vi "Команда обмена 5 (доп. команда) (SubVI).vi"(3 "Выстрелов до перемотки":u16=100, 7 "error in":errorcluster, 13 "номер мишени (id)":u16) -> (23 "Кластер параметров 15-ой команды":T1, 27 "error out":errorcluster)   [LabVIEW 2013]
doc: "Доп. команда - передача числа выстрелов до перемотки пленки"
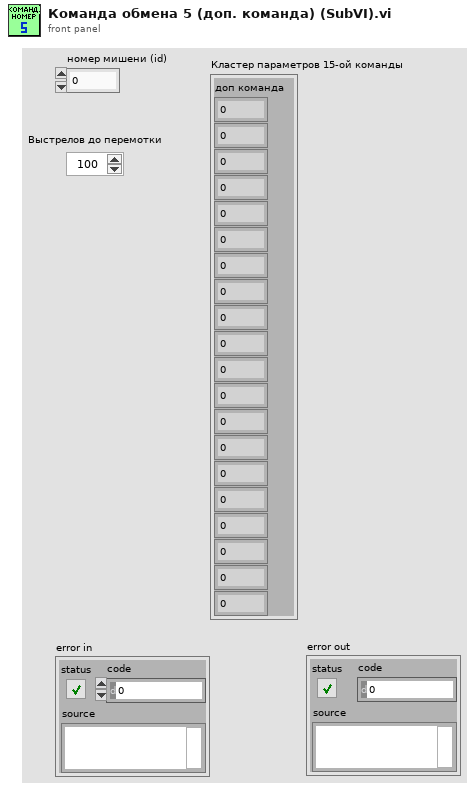
[diagram p1: front panel]
types:
  T1 = cluster{"доп команда":u8, u8, u8, u8, u8, u8, u8, u8, u8, u8, u8, u8, u8, u8, u8, u8, u8, u8, u8, u8}
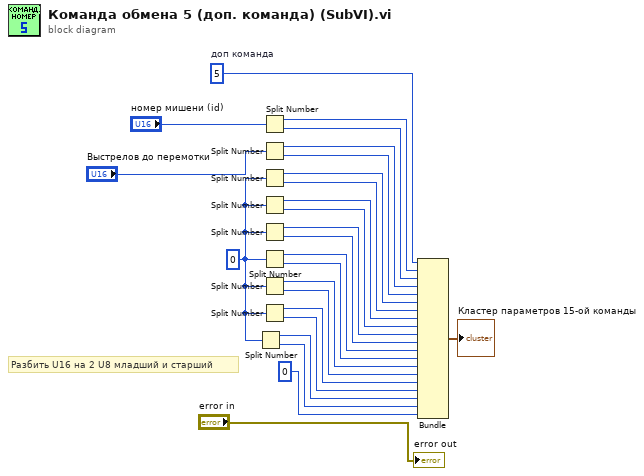
[diagram p0: block diagram]
diagram:
  w3 = u8 0
  w8 = u8 5  # доп команда
  # "Разбить U16 на 2 U8 младший и старший"
  n1 = Split Number(x=w3) -> (hi(x)=w23:u8, lo(x)=w24:u8)
  n2 = Split Number(x="номер мишени (id)") -> (hi(x)=w6:u8, lo(x)=w5:u8)
  n3 = Split Number(x="Выстрелов до перемотки") -> (hi(x)=w9:u8, lo(x)=w10:u8)
  n4 = Split Number(x=w3) -> (hi(x)=w11:u8, lo(x)=w12:u8)
  n5 = Split Number(x=w3) -> (hi(x)=w13:u8, lo(x)=w14:u8)
  n6 = Split Number(x=w3) -> (hi(x)=w15:u8, lo(x)=w16:u8)
  n7 = Split Number(x=w3) -> (hi(x)=w17:u8, lo(x)=w18:u8)
  n8 = Split Number(x=w3) -> (hi(x)=w19:u8, lo(x)=w20:u8)
  n9 = Split Number(x=w3) -> (hi(x)=w21:u8, lo(x)=w22:u8)
  n10 = Bundle("доп команда"=w8, w6, w5, w9, w10, w11, w12, w13, w14, w15, w16, w17, w18, w19, w20, w21, w22, w23, w24, u8 0) -> (→"Кластер параметров 15-ой команды":T1)  [unwired: 1 in]
  "error out" <- "error in"
